vi "Prepare Templating.vi"(8 "error in (no error)":errorcluster, 11 "BasicTemplater in":refnum<class "BasicTemplater.lvclass">) -> (0 "error out":errorcluster, 3 "BasicTemplater out":refnum<class "BasicTemplater.lvclass">)   [LabVIEW 2020, in "HTTP Server.lvlib" / "BasicTemplater.lvclass"]
uses:
  BasicTemplater.lvclass
  BasicTemplater.lvclass/BasicTemplater.ctl
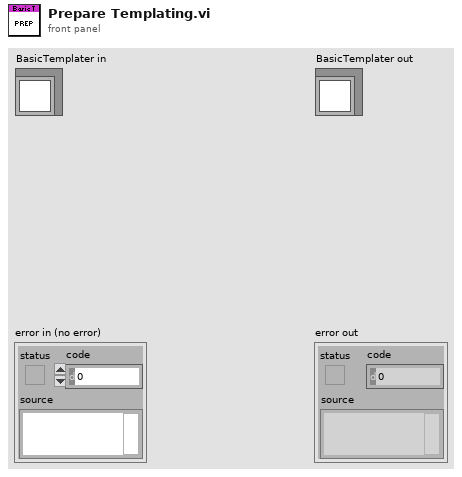
[diagram p1: front panel]
types:
  T1 = map{string, refnum<class "TemplateValueResolver.lvclass">}
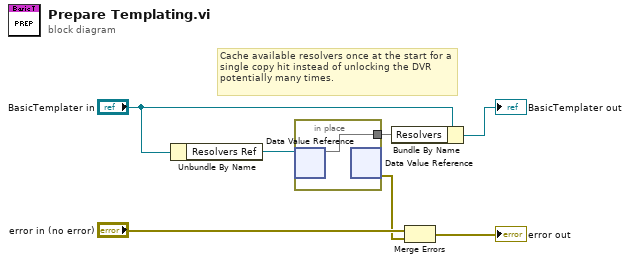
[diagram p0: block diagram]
diagram:
  # "Cache available resolvers once at the start for a single copy hit instead of unlocking the DVR potentially many times."
  n1 = Unbundle By Name("BasicTemplater in") -> ("Resolvers Ref"=w6:refnum<data-value>)
  n2 = in-place {
    in-place-border: [w8] -> w3
    n3 = in-place-dvr #1(w6) -> (w8:T1)  [unwired: 1 out]
    n4 = in-place-dvr #1() -> (w1:errorcluster)  [unwired: 1 in, 1 out]
  }
  n5 = Bundle By Name(cluster="BasicTemplater in", "Resolvers"=w3) -> (→"BasicTemplater out":refnum<class "BasicTemplater.lvclass">)
  n6 = Merge Errors("error in (no error)", w1) -> (→"error out":errorcluster)
